vi "LV86_Morph_Erosion.vi"(2 "Connectivity":enum16{"4", "6", "8"}(ring), 3 "Image in":T1 {"Dialogs" format="%.0b"}) -> (1 "Image out":T1 {"Dialogs" format="%.0b"})   [LabVIEW 2024]
doc: "This VI performs an erosion on the input image using the given <B>connectivity</B>. This typically shrinks features in binary images."
uses:
  <userlib>/ImageProcessing/QTLIB_2595_LV86/QT_Image.ctl
  <vilib>/Analysis/2dsp.llb/2D Convolution (DBL).vi
  <vilib>/Analysis/NI_AALPro.lvlib
panel:
  out "Initial Image":picture caption="new picture"
  out "Erosion":picture caption="new picture"
  # "This VI performs an erosion on the input image using \nthe given connectivity.  This typically shrinks \nfeatures in binary images."
  # "Initial Image"
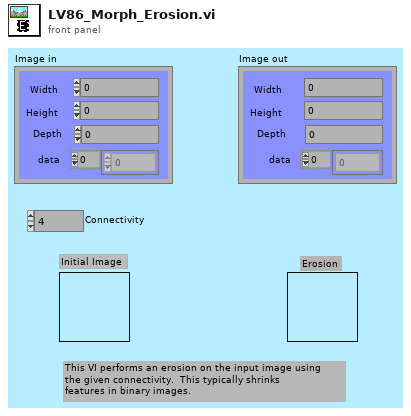
[diagram p1: front panel]
types:
  T1 = typedef "QT_Image.ctl" = cluster{"Width":i32, "Height":i32, "Depth":i32, "data":u8[], "Compressed data":u8[], "Color table":u32[], "Duration":i32, "Options":i32, "Timestamp":i32, "ID":i32, "Reserved":i32, "Dialogs":u32}
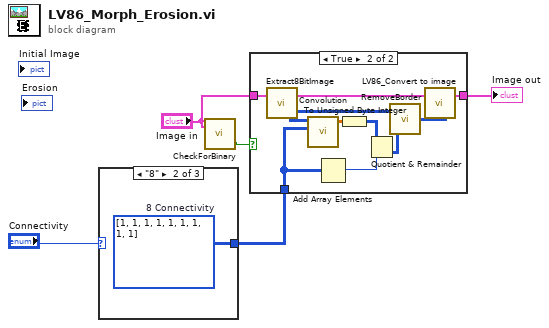
[diagram p0: block diagram]
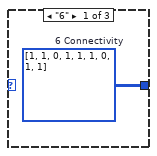
[diagram p3: hidden frame]
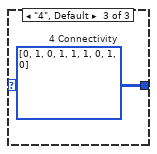
[diagram p4: hidden frame]
diagram:
  n1 = case shown="\"8\"" "Connectivity" {
    tunnel: [w6 w7 w8] -> w2
    frame "6" {
      w6 = u8[][] [[1, 1, 0], [1, 1, 1], [0, 1, 1]]  # 6 Connectivity
    }
    frame "8" {
      w7 = u8[][] [[1, 1, 1], [1, 1, 1], [1, 1, 1]]  # 8 Connectivity
    }
    frame "4", Default {
      w8 = u8[][] [[0, 1, 0], [1, 1, 1], [0, 1, 0]]  # 4 Connectivity
    }
  }
  n2 = call <userlib>:"CheckForBinary.vi"("Image in"="Image in") -> ("Success?"=w1:bool)  [unwired: 2 out]
  n3 = case shown="True" w1 {
    tunnel: "Image in" -> [w9 w18]
    tunnel: [w9 w17] -> w3
    tunnel: w2 -> [_ w16]
    frame False {
    }
    frame True {
      n4 = call <userlib>:"Extract8BitImage.vi"("Image in"=w18) -> ("Intensity Graph"=w11:u8[][], "Image out"=w19:T1)  [unwired: 1 in]
      n5 = call-poly <vilib>:"Convolution.vi"("Y"=w16, "X"=w11) -> ("X * Y"=w14:dbl[][])  [unwired: 2 in, 7 out]
      n6 = Add Array Elements(numeric array=w16) -> (sum=w15:u8)
      n7 = To Unsigned Byte Integer(number=w14) -> (unsigned 8bit integer=w13:u8[][])
      n8 = Quotient & Remainder(x=w13, y=w15) -> (floor(x/y)=w12:u8[][])  [unwired: 1 out]
      n9 = call <userlib>:"RemoveBorder.vi"("Larger Image"=w12, "Original Image"=w11) -> ("Subset"=w10:u8[][])
      n10 = call <userlib>:"LV86_Convert to image.vi"("Intensity Graph"=w10, "Image In"=w19) -> ("Image Out"=w17:T1)  [unwired: 1 in]
    }
  }
  "Image out" <- w3
